vi "Send (no data).vi"(6 "Reply to...":refnum<class "Send.lvclass">, 8 "error in (no error)":errorcluster, 10 "Label":string, 11 "MSR Parent in":refnum<class "Send.lvclass">) -> (0 "error out":errorcluster, 3 "MSR Parent out":refnum<class "Send.lvclass">)   [LabVIEW 2011, in "Messenging.lvlib" / "Send.lvclass"]
uses:
  Send.lvclass
  TextVarientMessage/MSG.lvclass
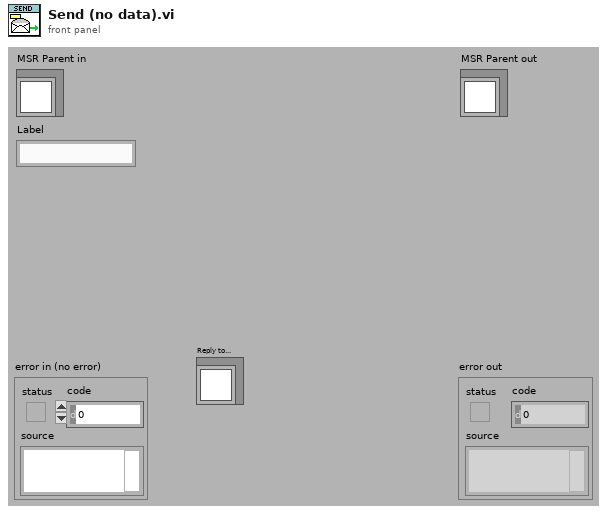
[diagram p1: front panel]
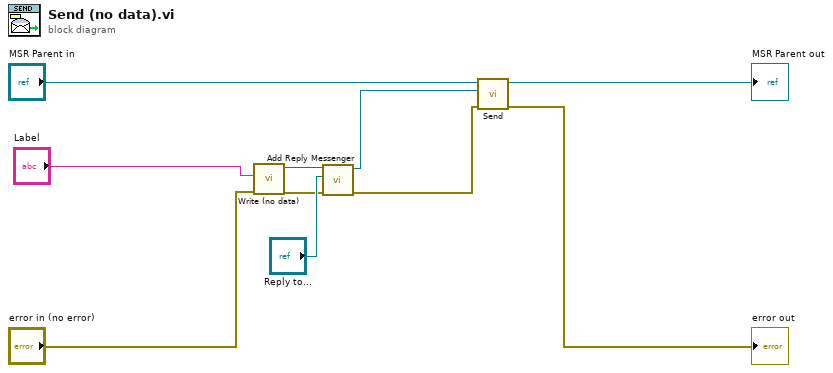
[diagram p0: block diagram]
diagram:
  n1 = call "Write (no data).vi"("error in (no error)"="error in (no error)", "Label"="Label") -> ("error out"=w3:errorcluster, "Message"=w5:refnum<class "MSG.lvclass">)  [unwired: 8 out]
  n2 = call "Add Reply Messenger.vi"("error in (no error)"=w3, "Reply to..."="Reply to...", "Message"=w5) -> ("error out"=w2:errorcluster, "Message"=w1:refnum<class "MSG.lvclass">)  [unwired: 7 out]
  n3 = call-dynamic "Send.vi"("error in (no error)"=w2, "Message"=w1, "MSR Parent in"="MSR Parent in") -> ("error out"=→"error out":errorcluster, "MSR Parent out"=→"MSR Parent out":refnum<class "Send.lvclass">)  [unwired: 7 out]
